vi "Create_New_Build.vi"(6 "buildSpecName":string, 7 "Programmatic? (false)":bool, 8 "error in (no error)":errorcluster, 9 "buildObject":T1, 10 "Destination Path":path, 11 "AB_DLL in":refnum<class "AB_DLL.lvclass">) -> (0 "error out":errorcluster, 3 "AB_DLL out":refnum<class "AB_DLL.lvclass">)   [LabVIEW 2020, in "AB_DLL.lvclass"]
uses:
  <vilib>/AppBuilder/AB_Classes/DLL/AB_DLL.lvclass
  <resource>/Framework/Providers/API/ItemRef.ctl
  <vilib>/AppBuilder/AB_TargetFileType.ctl
  <vilib>/AppBuilder/AB_Classes/DLL/AB_DLL.lvclass/AB_DLL.ctl
  <resource>/Framework/Providers/Common/provcom_StringGlobals.vi
  <vilib>/AppBuilder/AB_Classes/Application/AB_Application.lvclass
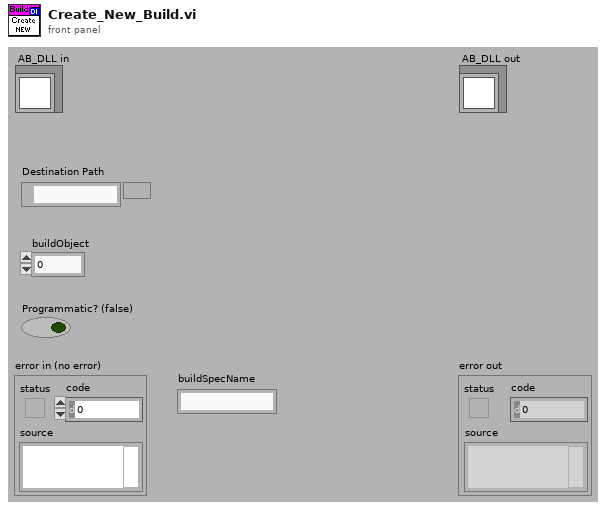
[diagram p1: front panel]
types:
  T1 = typedef "ItemRef.ctl" = u64
  T2 = typedef "AB_TargetFileType.ctl" = enum16{"EXE", "DLL", "RTEXE"}
  T3 = enum32{"invalid OS target", "Mac OS", "Windows 3.1", "Windows 95/NT", "Solaris 1", "Solaris 2", "HP-UX", "PowerMAX", "Linux", "Irix", "Rhapsody", "BeOS", "AIX", "OSF1", "VxWorks", "PharLap", "Carbon", "RTX", "Windows x64", "Linux x64", "Mac OS X x64"}
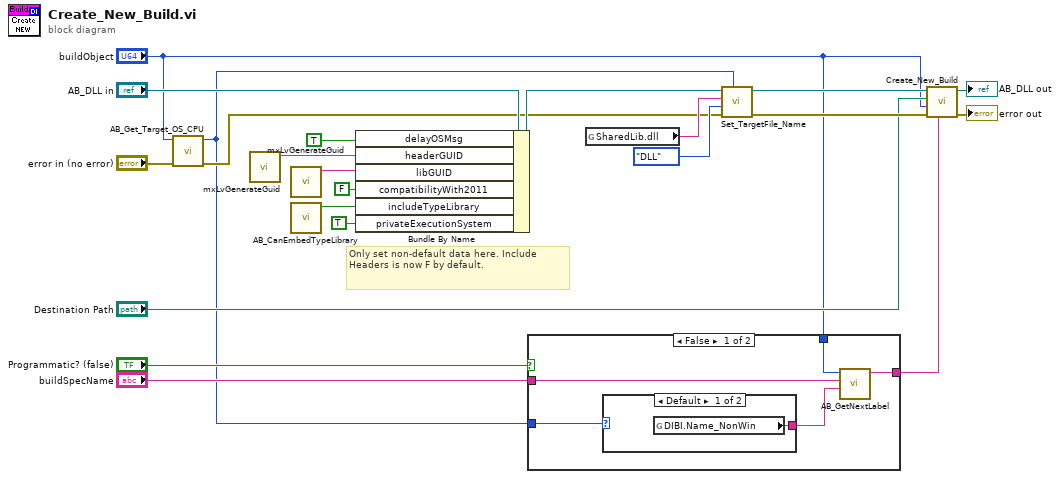
[diagram p0: block diagram]
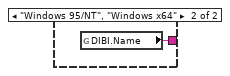
[diagram p2: hidden frame]
diagram:
  # "Only set non-default data here. Include Headers is now F by default."
  n1 = call <resource>:"AB_Get_Target_OS_CPU.vi"("error in (no error)"="error in (no error)", "Object"="buildObject") -> ("error out"=w4:errorcluster, "Target Operating System"=w3:T3)  [unwired: 7 in, 1 out]
  n2 = call <resource>:"mxLvGenerateGuid.vi"() -> ("Value"=w17:string)  [unwired: 1 in, 10 out]
  n3 = call <resource>:"mxLvGenerateGuid.vi"() -> ("Value"=w16:string)  [unwired: 1 in, 10 out]
  n4 = call <vilib>:"AB_CanEmbedTypeLibrary.vi"() -> ("Can embed type library?"=w2:bool)  [unwired: 10 in, 1 out]
  n5 = Bundle By Name(cluster="AB_DLL in", "delayOSMsg"=TRUE ("data.delayOSMsg"), "headerGUID"=w17, "libGUID"=w16, "compatibilityWith2011"=FALSE ("data.compatibilityWith2011"), "includeTypeLibrary"=w2, "privateExecutionSystem"=TRUE ("data.privateExecutionSystem")) -> (w12:refnum<class "AB_DLL.lvclass">)
  n6 = case shown="False" "Programmatic? (false)" {
    tunnel: "buildObject" -> [w24 _]
    tunnel: [w27 w30] -> w20
    tunnel: "buildSpecName" -> [w25 w30]
    tunnel: w3 -> [w23 _]
    frame False {
      n7 = case shown="Default" w23 {
        tunnel: [w28 w29] -> w26
        frame Default {
          n8 = global read "provcom_StringGlobals.vi" "DIBI.Name_NonWin"() -> (w28:string)
        }
        frame "Windows 95/NT", "Windows x64" {
          n9 = global read "provcom_StringGlobals.vi" "DIBI.Name"() -> (w29:string)
        }
      }
      n10 = call <vilib>:"AB_GetNextLabel.vi"("default name"=w26, "supplied name"=w25, "buildObject"=w24) -> ("New label"=w27:string)  [unwired: 2 in, 6 out]
    }
    frame True {
    }
  }
  n11 = global read "provcom_StringGlobals.vi" "SharedLib.dll"() -> (w14:string)
  n12 = call-dynamic "Set_TargetFile_Name.vi"("Target Operating System"=w3, "error in (no error)"=w4, "Target file type"=AB_TargetFileType."DLL" ("Build type"), "Target file name"=w14, "AB_Targetfile in"=w12) -> ("error out"=w10:errorcluster, "AB_Targetfile out"=w11:refnum<class "AB_DLL.lvclass">)  [unwired: 5 in]
  n13 = call-parent "Create_New_Build.vi"("buildSpecName"=w20, "error in (no error)"=w10, "buildObject"="buildObject", "Destination Path"="Destination Path", "AB_Application in"=w11) -> ("error out"=→"error out":errorcluster, "AB_Application out"=→"AB_DLL out":refnum<class "AB_DLL.lvclass">)  [unwired: 1 in, 4 out]
